vi "Get primes less or equal to x.vi"(8 "error in (no error)":errorcluster, 11 "x = end":i32=1000) -> (0 "error out":errorcluster, 2 "Number of primes":i32, 3 "Primes":i32[](array[numeric]))   [LabVIEW 2021, in "Numeric Utilities.lvlib"]
uses:
  Numeric Utilities.lvlib
  Named Timers/Named Timers.lvlib
panel:
  out "Loop iteration":i32
  out "Execution time (s)":dbl
  in  "Dev: Stop Early":bool
  # "Input\nInputs to the VI"
  # "Development\ncontrols/indicators useful for development and testing, but which are not outputs of the VI"
  # "Output\nOutputs of the VI"
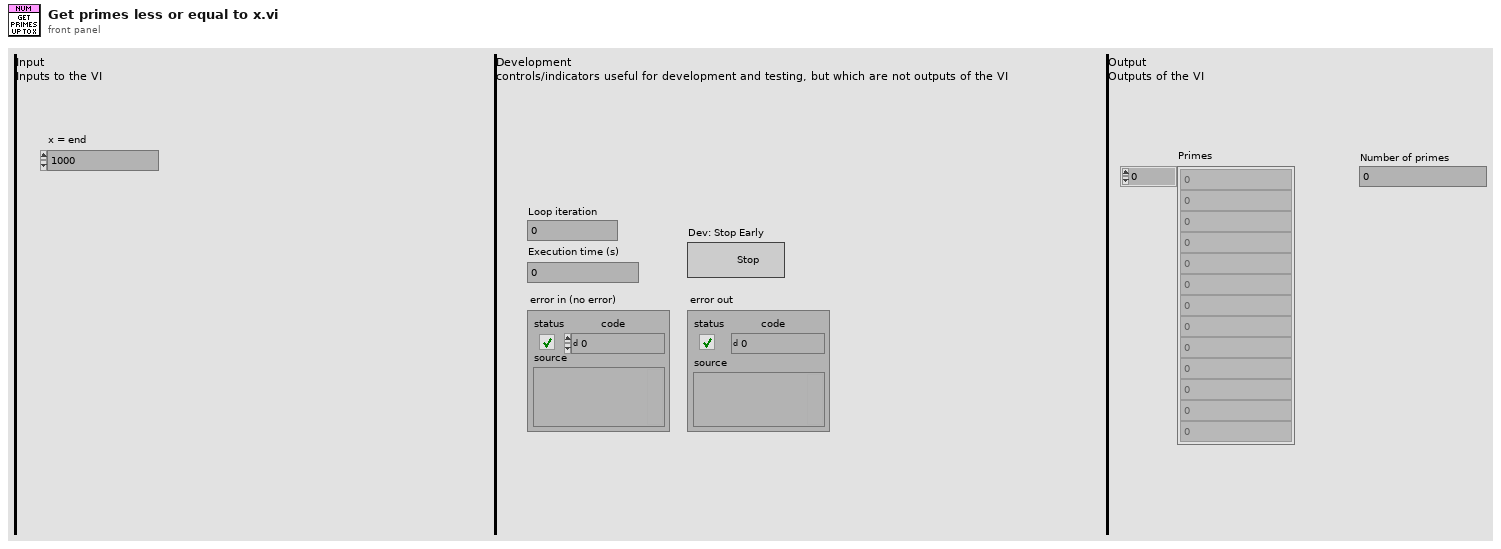
[diagram p1: front panel]
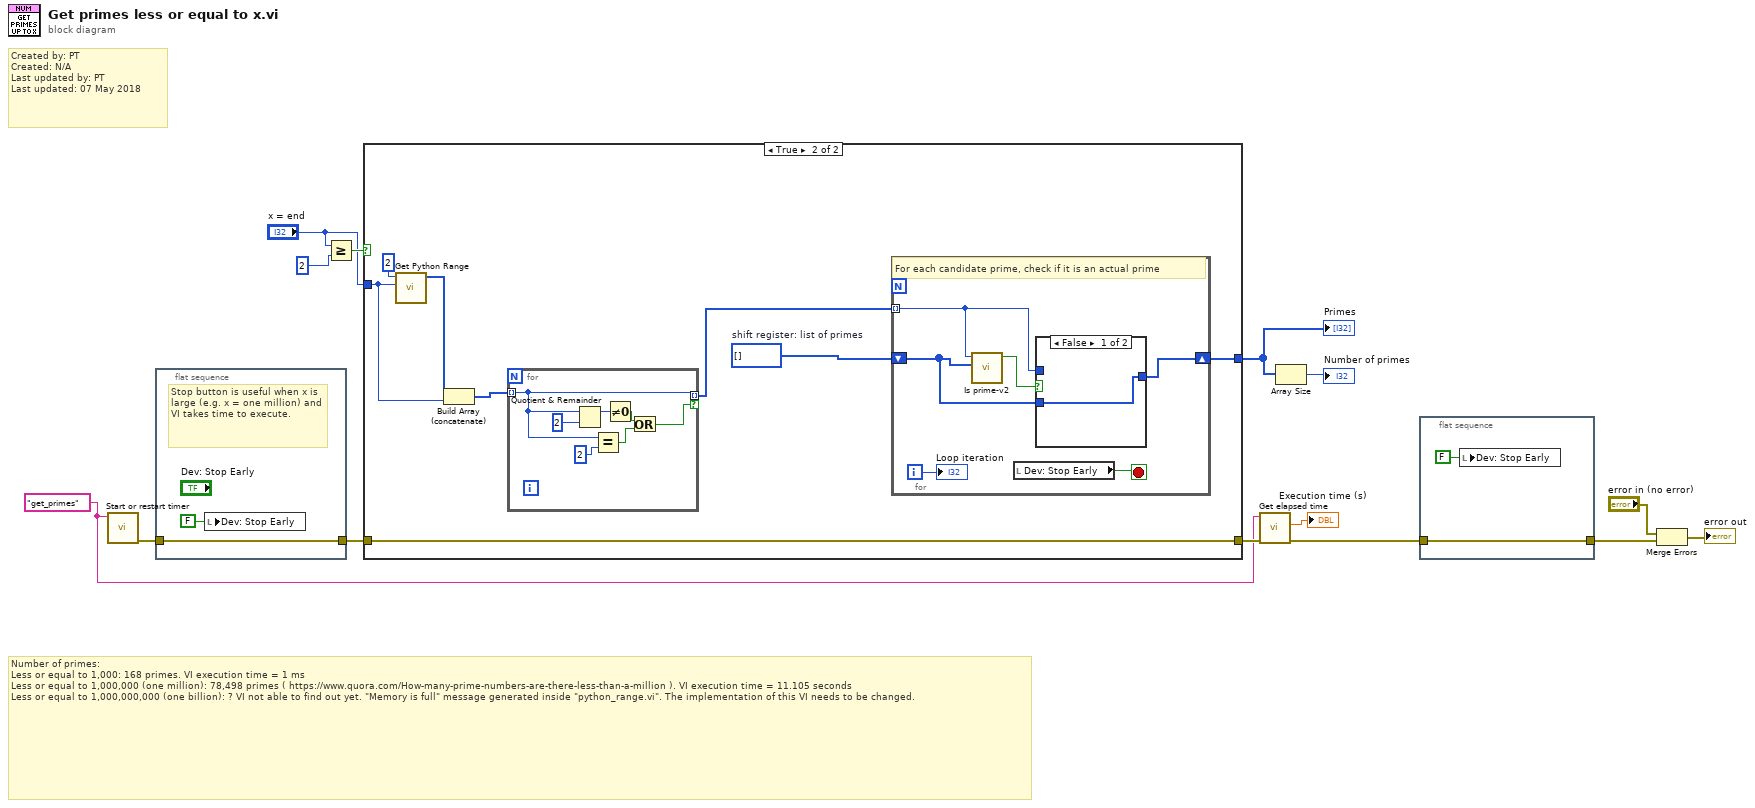
[diagram p0: block diagram]
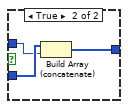
[diagram p3: hidden frame]
diagram:
  w9 = "get_primes"
  # "Number of primes:\nLess or equal to 1,000: 168 primes. VI execution time = 1 ms\nLess or equal to 1,000,000 (one million): 78,498 primes ( https://www.quora.com/How-many-prime-numbers-are-there-less-than-a-million ). VI execution time = 11.105 seconds\nLess or equal to 1,000,000,000 (one billion): ? VI not able to find out yet. \"Memory is full\" message generated inside \"python_range.vi\". The implementation of this VI needs to be changed."
  # "Created by: PT\nCreated: N/A\nLast updated by: PT\nLast updated: 07 May 2018"
  n1 = call "Start or restart timer.vi"("Timer name"=w9) -> ("error out"=w13:errorcluster)  [unwired: 10 in]
  n2 = flat-sequence {
    tunnel: w13 -> [w15]
    tunnel: [w15] -> w12
    frame #0 {
      # "Stop button is useful when x is large (e.g. x = one million) and VI takes time to execute."
      n3 = local write "Dev: Stop Early"(FALSE ("Stop Button")) -> ()
    }
  }
  n4 = Greater Or Equal?(x="x = end", y=2) -> (x >= y?=w14:bool)
  n5 = case shown="True" w14 {
    tunnel: "x = end" -> [_ w20]
    tunnel: [_ w25] -> w4
    tunnel: w12 -> [w17 w22]
    tunnel: [w17 w22] -> w10
    frame False {
      # "x = 0 or x = 1; no primes between 0 and x"
    }
    frame True {
      w18 = i32[] []  # shift register: list of primes
      n6 = call "Get Python Range.vi"("stop"=w20, "start"=2) -> ("range"=w24:i32[])  [unwired: 8 in, 1 out]
      n7 = Build Array (concatenate)(w24, w20) -> (w21:i32[])
      n8 = for {
        tunnel: w21 -> [w36] mode=indexing
        tunnel: [w36] -> w23 mode=indexing if=w40
        n9 = Quotient & Remainder(x=w36, y=2) -> (x-y*floor(x/y)=w39:i32)  [unwired: 1 out]
        n10 = Equal?(x=w36, y=2) -> (x = y?=w41:bool)
        n11 = Not Equal To 0?(x=w39) -> (x != 0?=w37:bool)
        n12 = Or(x=w37, y=w41) -> (x .or. y?=w40:bool)
      }
      n13 = for {
        tunnel: w23 -> [w30] mode=indexing
        shift-right: [w27] -> w25
        shift-left: w18 -> [w28]
        i -> [w26]
        stop <- w29 stop-if-true
        # "For each candidate prime, check if it is an actual prime"
        n14 = call "Is prime-v2.vi"("List of all prime numbers smaller than x"=w28, "x"=w30) -> ("T = is prime"=w31:bool)  [unwired: 8 in, 1 out]
        n15 = local read "Dev: Stop Early"() -> (w29:bool)
        n16 = case shown="False" w31 {
          tunnel: w30 -> [_ w34]
          tunnel: w28 -> [w32 w35]
          tunnel: [w32 w33] -> w27
          frame False {
          }
          frame True {
            n17 = Build Array (concatenate)(w35, w34) -> (w33:i32[])
          }
        }
        "Loop iteration" <- w26
      }
    }
  }
  "Primes" <- w4
  n18 = call "Get elapsed time.vi"("error in (no error)"=w10, "Timer name"=w9) -> ("error out"=w8:errorcluster, "Elapsed time (s)"=→"Execution time (s)":dbl)  [unwired: 6 in, 2 out]
  n19 = Array Size(array=w4) -> (size(s)=→"Number of primes":i32)
  n20 = flat-sequence {
    tunnel: w8 -> [w43]
    tunnel: [w43] -> w1
    frame #0 {
      n21 = local write "Dev: Stop Early"(FALSE ("Stop Button")) -> ()
    }
  }
  n22 = Merge Errors("error in (no error)", w1) -> (→"error out":errorcluster)
